vi "InRange.vi"(9 "Min":dbl, 10 "Value":dbl, 11 "Max":dbl) -> (3 "Boolean":bool)   [LabVIEW 2017]
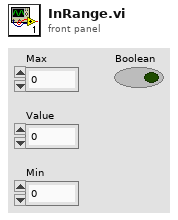
[diagram p1: front panel]
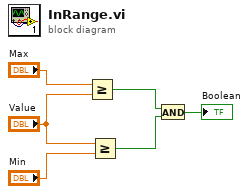
[diagram p0: block diagram]
diagram:
  n1 = Greater Or Equal?(x="Max", y="Value") -> (x >= y?=w4:bool)
  n2 = Greater Or Equal?(x="Value", y="Min") -> (x >= y?=w5:bool)
  n3 = And(x=w4, y=w5) -> (x .and. y?=→"Boolean":bool)
